vi "DBValueToDBMessage.vi"(11 "AValue":string) -> (3 "DBMessage":T1 {"BRS" items=["No BRS", "BRS"]; "ID" format="%.0x"; "Type" items=["cftStdCAN", "cftExtCAN", "cftJ1939", "cftStdCANFD", "cftExtCANFD"]})   [LabVIEW 2014]
uses:
  Typedef/DBMessage.ctl
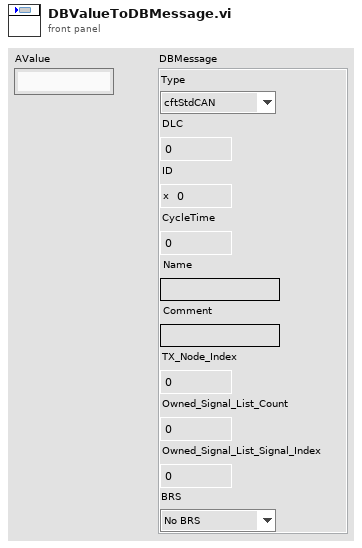
[diagram p1: front panel]
types:
  T1 = typedef "DBMessage.ctl" = cluster{"Type":u16, "DLC":i32, "ID":i32, "CycleTime":dbl, "Name":string, "Comment":string, "TX_Node_Index":i32, "Owned_Signal_List_Count ":i32, "Owned_Signal_List_Signal_Index":i32, "BRS":i32}
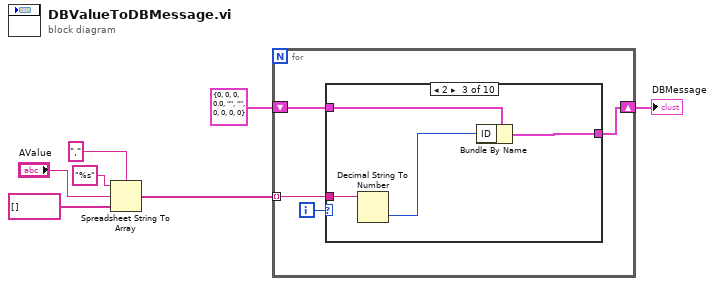
[diagram p0: block diagram]
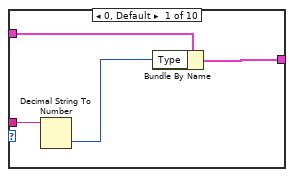
[diagram p2: hidden frame]
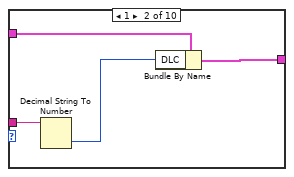
[diagram p3: hidden frame]
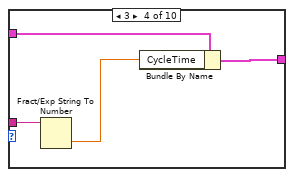
[diagram p4: hidden frame]
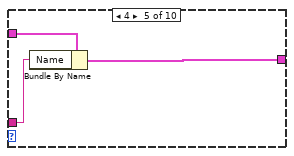
[diagram p5: hidden frame]
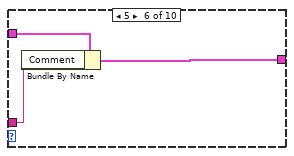
[diagram p6: hidden frame]
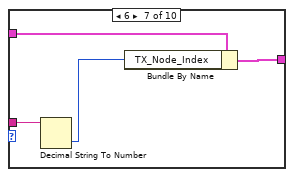
[diagram p7: hidden frame]
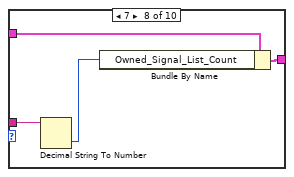
[diagram p8: hidden frame]
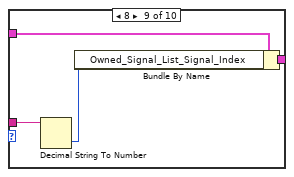
[diagram p9: hidden frame]
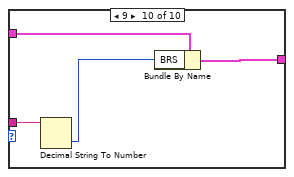
[diagram p10: hidden frame]
diagram:
  n1 = Spreadsheet String To Array(delimiter (Tab)=",", format string="%s", spreadsheet string="AValue", array type (2D Dbl)=string[] []) -> (array=w1:string[])
  n2 = for {
    tunnel: w1 -> [w10] mode=indexing
    shift-right: [w8] -> w7
    shift-left: T1 {"Type"=0, "DLC"=0, "ID"=0, "CycleTime"=0.0, "Name"="", "Comment"="", "TX_Node_Index"=0, "Owned_Signal_List_Count "=0, "Owned_Signal_List_Signal_Index"=0, "BRS"=0} ("DBMessage") -> [w9]
    i -> [w11]
    n3 = case shown="2" w11 {
      tunnel: w10 -> [w15 w19 w23 w27 w28 w31 w35 w39 w43 w47]
      tunnel: w9 -> [w14 w18 w22 w26 w30 w33 w37 w41 w45 w49]
      tunnel: [w12 w16 w20 w24 w29 w32 w36 w40 w44 w48] -> w8
      frame 0, Default {
        n4 = Decimal String To Number(string=w15) -> (number=w13:i32)  [unwired: 2 in, 1 out]
        n5 = Bundle By Name(cluster=w14, "Type"=w13) -> (w12:T1)
      }
      frame 1 {
        n6 = Decimal String To Number(string=w19) -> (number=w17:i32)  [unwired: 2 in, 1 out]
        n7 = Bundle By Name(cluster=w18, "DLC"=w17) -> (w16:T1)
      }
      frame 2 {
        n8 = Decimal String To Number(string=w23) -> (number=w21:i32)  [unwired: 2 in, 1 out]
        n9 = Bundle By Name(cluster=w22, "ID"=w21) -> (w20:T1)
      }
      frame 3 {
        n10 = Fract/Exp String To Number(string=w27) -> (number=w25:dbl)  [unwired: 3 in, 1 out]
        n11 = Bundle By Name(cluster=w26, "CycleTime"=w25) -> (w24:T1)
      }
      frame 4 {
        n12 = Bundle By Name(cluster=w30, "Name"=w28) -> (w29:T1)
      }
      frame 5 {
        n13 = Bundle By Name(cluster=w33, "Comment"=w31) -> (w32:T1)
      }
      frame 6 {
        n14 = Decimal String To Number(string=w35) -> (number=w34:i32)  [unwired: 2 in, 1 out]
        n15 = Bundle By Name(cluster=w37, "TX_Node_Index"=w34) -> (w36:T1)
      }
      frame 7 {
        n16 = Decimal String To Number(string=w39) -> (number=w38:i32)  [unwired: 2 in, 1 out]
        n17 = Bundle By Name(cluster=w41, "Owned_Signal_List_Count"=w38) -> (w40:T1)
      }
      frame 8 {
        n18 = Decimal String To Number(string=w43) -> (number=w42:i32)  [unwired: 2 in, 1 out]
        n19 = Bundle By Name(cluster=w45, "Owned_Signal_List_Signal_Index"=w42) -> (w44:T1)
      }
      frame 9 {
        n20 = Decimal String To Number(string=w47) -> (number=w46:i32)  [unwired: 2 in, 1 out]
        n21 = Bundle By Name(cluster=w49, "BRS"=w46) -> (w48:T1)
      }
    }
  }
  "DBMessage" <- w7
